vi "Test Quantum Design.vi"() -> ()   [LabVIEW 2018]
uses:
  Quantum Design Driver/Quantum Desing Configuration.ctl
  Quantum Design Driver/Quantum Design Driver.lvclass
panel:
  out "Waveform Chart":dbl[](graph)
  in  "Stop Button":bool
  in  "Update period":dbl
  in  "Quantum Desing Configuration":T1={"Address"="127.0.0.1", "Instrument type"=0, "Remote"=FALSE, "Temperature"=FALSE, "Field"=FALSE} {"Instrument type" items=["PPMS", "VersaLab", "DynaCool", "SVSM"]}
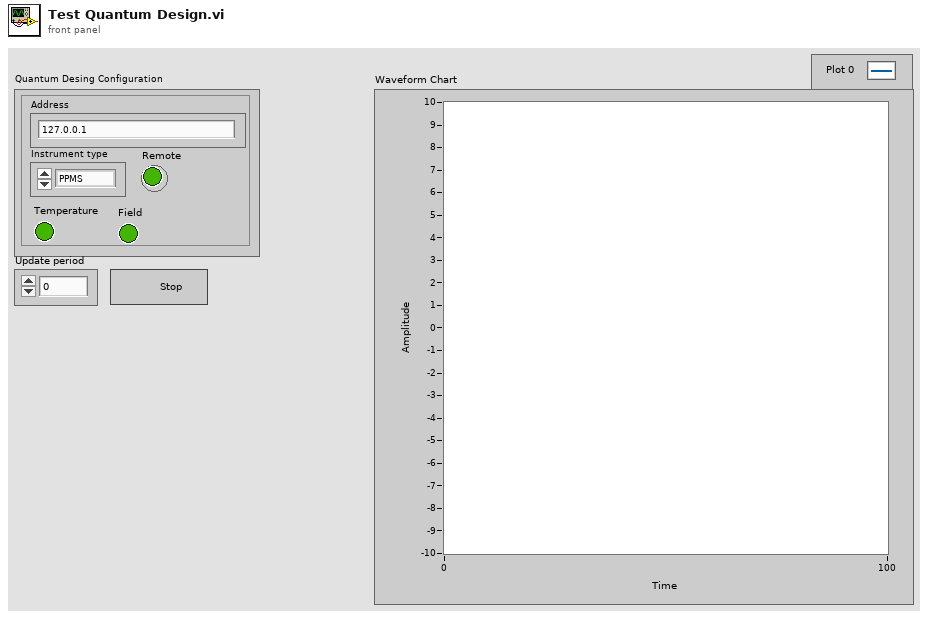
[diagram p1: front panel]
types:
  T1 = typedef "Quantum Desing Configuration.ctl" = cluster{"Address":string, "Instrument type":u16, "Remote":bool, "Temperature":bool, "Field":bool}
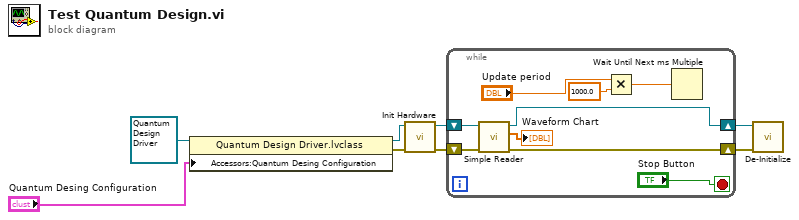
[diagram p0: block diagram]
diagram:
  n1 = property class="Quantum Design Driver.lvclass"(reference=refnum<class "Quantum Design Driver.lvclass"> refnum ("Quantum Design Driver.lvclass"), "Accessors:Quantum Desing Configuration"="Quantum Desing Configuration") -> (reference out=w7:refnum<class "Quantum Design Driver.lvclass">, error out=w5:errorcluster)  [unwired: 1 in]
  n2 = call-dynamic "Init Hardware.vi"("error in (no error)"=w5, "Quantum Design Driver in"=w7) -> ("error out"=w4:errorcluster, "Quantum Design Driver out"=w3:refnum<class "Quantum Design Driver.lvclass">)  [unwired: 8 in]
  n3 = while {
    shift-right: [w14] -> w1
    shift-left: w4 -> [w16]
    shift-right: [w15] -> w2
    shift-left: w3 -> [w17]
    stop <- "Stop Button" stop-if-true
    n4 = call-dynamic "Simple Reader.vi"("error in (no error)"=w16, "Quantum Design Driver in"=w17) -> ("error out"=w14:errorcluster, "Signals"=→"Waveform Chart":dbl[], "Quantum Design Driver out"=w15:refnum<class "Quantum Design Driver.lvclass">)  [unwired: 7 in]
    n5 = Multiply(x="Update period", y=1000.0) -> (x*y=w12:dbl)
    n6 = Wait Until Next ms Multiple(millisecond multiple=w12) -> ()  [unwired: 1 out]
  }
  n7 = call-dynamic "De-Initialize.vi"("error in (no error)"=w1, "Quantum Design Driver in"=w2) -> ()  [unwired: 8 in, 2 out]
